vi "Timer data class VI - retrieve enum state.vi"(8 "error in (no error)":errorcluster, 11 "Timer in":refnum<class "Timer.lvclass">) -> (0 "error out":errorcluster, 2 "State":T1, 3 "Timer out":refnum<class "Timer.lvclass">)   [LabVIEW 2010, in "Timer.lvclass"]
uses:
  Timer.lvclass
  Controls/Timing Control.ctl
  Timer.lvclass/Timer.ctl
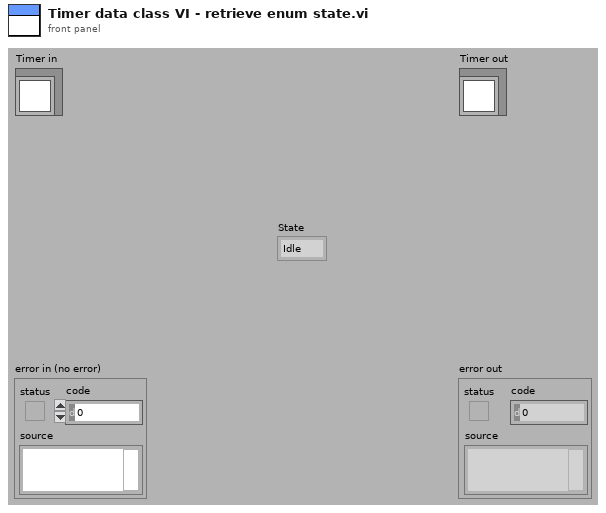
[diagram p1: front panel]
types:
  T1 = typedef "Timing Control.ctl" = enum16{"Idle", "Start", "Continue", "Reset"}
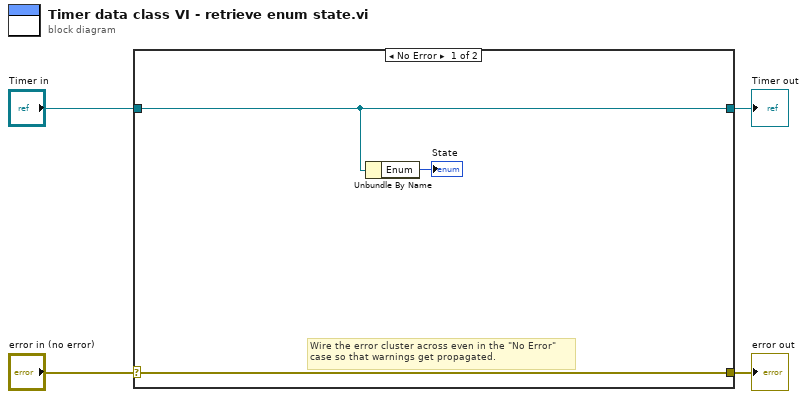
[diagram p0: block diagram]
diagram:
  n1 = case shown="No Error" "error in (no error)" {
    selector: "error in (no error)" -> [w7 w9]
    tunnel: [w7 w9] -> w3
    tunnel: [w6 w8] -> w1
    tunnel: "Timer in" -> [w6 w8]
    frame No Error {
      # "Wire the error cluster across even in the \"No Error\"\ncase so that warnings get propagated."
      n2 = Unbundle By Name(w6) -> ("Enum"=→"State":T1)
    }
    frame Error {
    }
  }
  "error out" <- w3
  "Timer out" <- w1
